vi "GetQueueMessageStatus.vi"(8 "error in":errorcluster, 10 "return elements? (F)":bool, 11 "message ref in":refnum<class "CLM_LocalMessage_Queue.lvclass">) -> (0 "error out":errorcluster, 1 "# pending insert":i32, 2 "# pending remove":i32, 3 "message ref out":refnum<class "CLM_LocalMessage_Queue.lvclass">, 4 "# elements in queue":i32, 5 "queue name":string, 6 "elements":T1[](array[typedef]), 7 "max queue size":i32)   [LabVIEW 2013, in "CLM_LocalMessage_Queue.lvclass"]
uses:
  CLM_LocalMessage_Queue.lvclass
  LocalMessage/Message.ctl
  CLM_LocalMessage_Queue.lvclass/CLM_LocalMessage_Queue.ctl
  LocalMessage/CLM_LocalMessage.lvclass
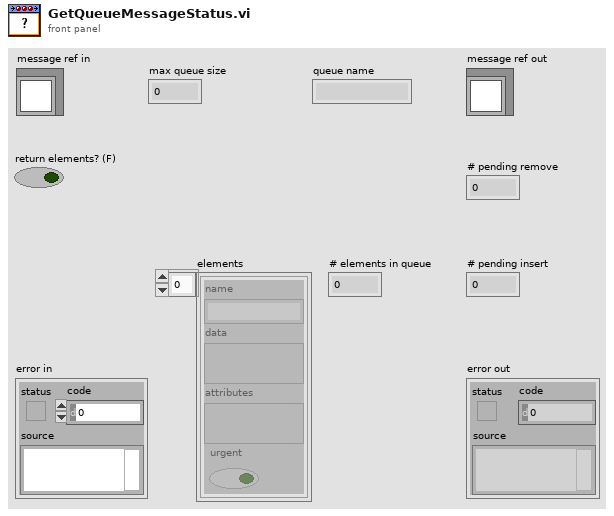
[diagram p1: front panel]
types:
  T1 = typedef "CLM_LocalMessage.lvclass/Message.ctl" = cluster{"name":string, "data":variant, "attributes":variant, "urgent":bool}
  T2 = typedef "CLM_LocalMessage_Queue.lvclass/MessageQueue.ctl" = refnum<queue>
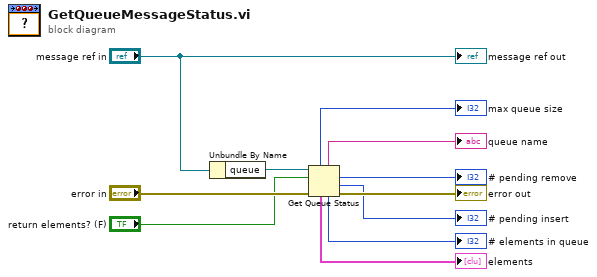
[diagram p0: block diagram]
diagram:
  n1 = Unbundle By Name("message ref in") -> ("queue"=w10:T2)
  n2 = Get Queue Status(queue=w10, return elements? (F)="return elements? (F)", error in (no error)="error in") -> (queue name=→"queue name":string, max queue size=→"max queue size":i32, # pending remove=→"# pending remove":i32, # pending insert=→"# pending insert":i32, error out=→"error out":errorcluster, # elements in queue=→"# elements in queue":i32, elements=→"elements":T1[])  [unwired: 1 out]
  "message ref out" <- "message ref in"
